vi "Init Channel Write Single.vi"(8 "error in":errorcluster, 9 "Channel Index":i32=1, 10 "Init Channels STS":i32, 11 "Init Channels In":refnum<class "Init Channels.lvclass">) -> (0 "error out":errorcluster, 3 "Init Channels Out":refnum<class "Init Channels.lvclass">)   [LabVIEW 2023, in "Init Channels.lvclass"]
uses:
  Init Channels.lvclass
  <vilib>/ADAS Replay HIL/Channels/Tag Wrapper/Tag Wrapper.lvlib
  <vilib>/ADAS Replay HIL/Channels/Tag Wrapper/Polymorphic/Write Channel (I32).vi
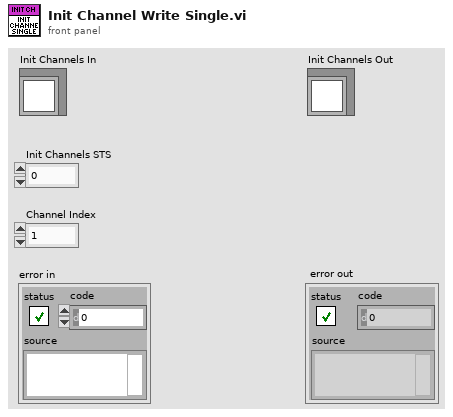
[diagram p1: front panel]
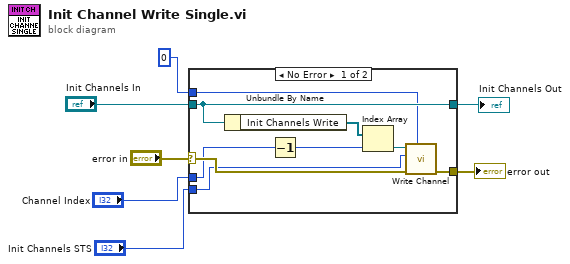
[diagram p0: block diagram]
diagram:
  n1 = case shown="No Error" "error in" {
    selector: "error in" -> [w16 w17]
    tunnel: [w15 w17] -> w6
    tunnel: [w12 w18] -> w1
    tunnel: "Init Channels In" -> [w12 w18]
    tunnel: "Channel Index" -> [w14 _]
    tunnel: "Init Channels STS" -> [w9 _]
    tunnel: 0 ("Timeout (ms)") -> [w8 _]
    frame No Error {
      n2 = Unbundle By Name(w12) -> ("Init Channels Write"=w11:refnum<k21>[])
      n3 = Decrement(x=w14) -> (x-1=w13:i32)
      n4 = Index Array(array=w11, index=w13) -> (element=w10:refnum<k21>)
      n5 = call-poly <vilib>:"Write Channel.vi"("Timeout (ms)"=w8, "error in"=w16, "Value to Write"=w9, "ADAS HIL Channel in"=w10) -> ("error out"=w15:errorcluster)  [unwired: 5 in, 2 out]
    }
    frame Error {
    }
  }
  "error out" <- w6
  "Init Channels Out" <- w1
